vi "Generate Waveform.vi"(6 "Spl Info":cluster{"Fs":dbl, "#s":dbl}, 8 "error in":errorcluster, 9 "Wave Amp":dbl, 10 "Wave Freq":dbl, 11 "Wave Type":T1=enum."Sine" caption="Signal Type") -> (0 "error out":errorcluster, 3 "Y":waveform(dbl))   [LabVIEW 2014]
uses:
  Ctls/Wave Type.ctl
  <vilib>/measure/NI_MABase.lvlib
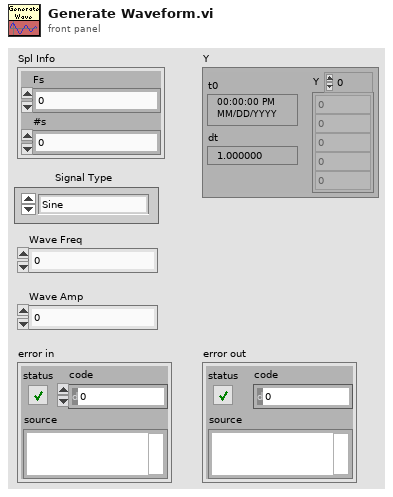
[diagram p1: front panel]
types:
  T1 = typedef "Wave Type.ctl" = enum16{"Bimodal Sine Wave", "Uniform White Noise", "Sine", "Square", "Ramp", "White Noise", "Square with Noise", "Sine with Noise"}
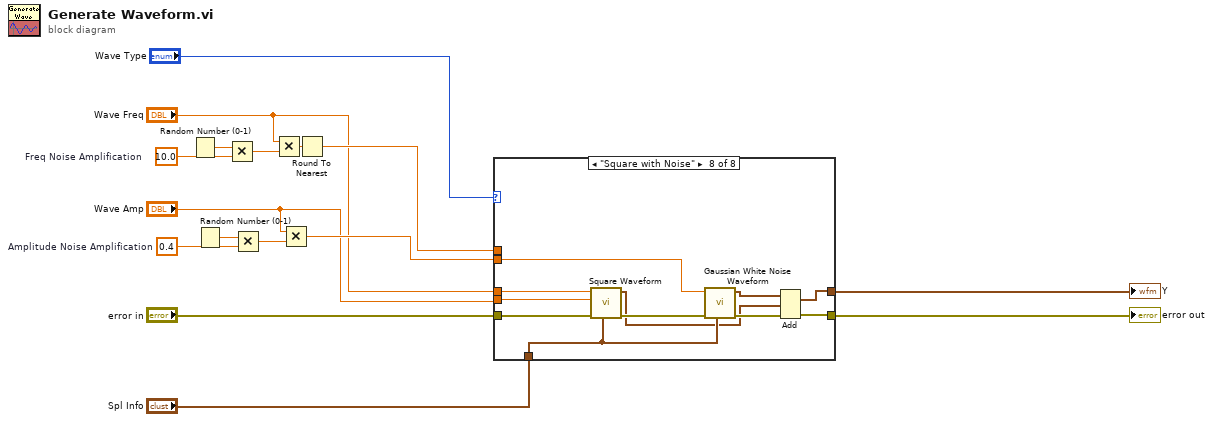
[diagram p0: block diagram]
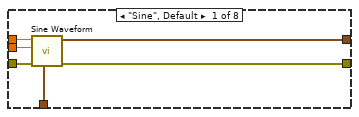
[diagram p2: hidden frame]
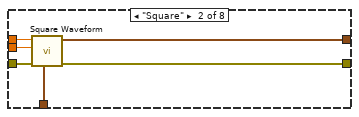
[diagram p3: hidden frame]
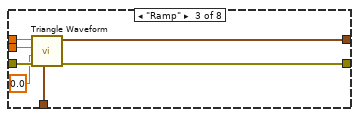
[diagram p4: hidden frame]
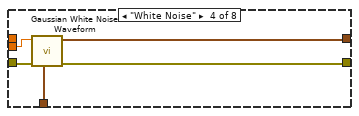
[diagram p5: hidden frame]
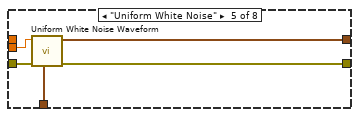
[diagram p6: hidden frame]
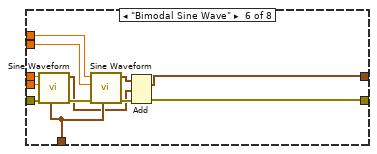
[diagram p7: hidden frame]
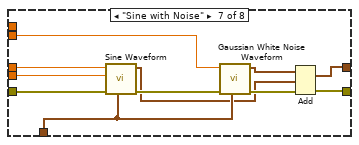
[diagram p8: hidden frame]
diagram:
  w14 = 0.4  # Amplitude Noise Amplification
  w13 = 10.0  # Freq Noise Amplification
  n1 = Random Number (0-1)() -> (number: 0 to 1=w12:dbl)
  n2 = Random Number (0-1)() -> (number: 0 to 1=w11:dbl)
  n3 = Multiply(x=w12, y=w13) -> (x*y=w15:dbl)
  n4 = Multiply(x=w11, y=w14) -> (x*y=w16:dbl)
  n5 = Multiply(x="Wave Freq", y=w15) -> (x*y=w7:dbl)
  n6 = Multiply(x="Wave Amp", y=w16) -> (x*y=w10:dbl)
  n7 = Round To Nearest(number=w7) -> (nearest integer value=w8:dbl)
  n8 = case shown="\"Square with Noise\"" "Wave Type" {
    tunnel: "Spl Info" -> [w22 w23 w30 w39 w45 w54 w65 w76]
    tunnel: "Wave Freq" -> [w21 w25 w32 _ _ w57 w68 w79]
    tunnel: "Wave Amp" -> [w20 w24 w31 w36 w41 w56 w67 w78]
    tunnel: "error in" -> [w19 w28 w35 w37 w44 w55 w66 w77]
    tunnel: [w18 w27 w34 w40 w43 w51 w62 w73] -> w4
    tunnel: [w17 w26 w33 w38 w42 w50 w61 w72] -> w5
    tunnel: w8 -> [_ _ _ _ _ w46 _ _]
    tunnel: w10 -> [_ _ _ _ _ w47 w58 w69]
    frame "Sine", Default {
      n9 = call <vilib>:"Sine Waveform.vi"("sampling info"=w22, "error in (no error)"=w19, "amplitude"=w20, "frequency"=w21) -> ("error out"=w18:errorcluster, "signal out"=w17:waveform(dbl))  [unwired: 6 in]
    }
    frame "Square" {
      n10 = call <vilib>:"Square Waveform.vi"("sampling info"=w23, "error in (no error)"=w28, "amplitude"=w24, "frequency"=w25) -> ("error out"=w27:errorcluster, "signal out"=w26:waveform(dbl))  [unwired: 6 in]
    }
    frame "Ramp" {
      n11 = call <vilib>:"Triangle Waveform.vi"("sampling info"=w30, "error in (no error)"=w35, "phase"=0.0, "amplitude"=w31, "frequency"=w32) -> ("error out"=w34:errorcluster, "signal out"=w33:waveform(dbl))  [unwired: 5 in]
    }
    frame "White Noise" {
      n12 = call <vilib>:"Gaussian White Noise Waveform.vi"("sampling info"=w39, "error in (no error)"=w37, "standard deviation"=w36) -> ("error out"=w40:errorcluster, "signal out"=w38:waveform(dbl))  [unwired: 7 in]
    }
    frame "Uniform White Noise" {
      n13 = call <vilib>:"Uniform White Noise Waveform.vi"("sampling info"=w45, "error in (no error)"=w44, "amplitude"=w41) -> ("error out"=w43:errorcluster, "signal out"=w42:waveform(dbl))  [unwired: 7 in]
    }
    frame "Bimodal Sine Wave" {
      n14 = call <vilib>:"Sine Waveform.vi"("sampling info"=w54, "error in (no error)"=w55, "amplitude"=w56, "frequency"=w57) -> ("error out"=w53:errorcluster, "signal out"=w48:waveform(dbl))  [unwired: 6 in]
      n15 = call <vilib>:"Sine Waveform.vi"("sampling info"=w54, "error in (no error)"=w53, "amplitude"=w47, "frequency"=w46) -> ("error out"=w52:errorcluster, "signal out"=w49:waveform(dbl))  [unwired: 6 in]
      n16 = Add(1:w48, 2:w49, 4:w52) -> (0:w50:waveform(dbl), 3:w51:errorcluster)
    }
    frame "Sine with Noise" {
      n17 = call <vilib>:"Sine Waveform.vi"("sampling info"=w65, "error in (no error)"=w66, "amplitude"=w67, "frequency"=w68) -> ("error out"=w64:errorcluster, "signal out"=w59:waveform(dbl))  [unwired: 6 in]
      n18 = call <vilib>:"Gaussian White Noise Waveform.vi"("sampling info"=w65, "error in (no error)"=w64, "standard deviation"=w58) -> ("error out"=w63:errorcluster, "signal out"=w60:waveform(dbl))  [unwired: 7 in]
      n19 = Add(1:w59, 2:w60, 4:w63) -> (0:w61:waveform(dbl), 3:w62:errorcluster)
    }
    frame "Square with Noise" {
      n20 = call <vilib>:"Square Waveform.vi"("sampling info"=w76, "error in (no error)"=w77, "amplitude"=w78, "frequency"=w79) -> ("error out"=w75:errorcluster, "signal out"=w70:waveform(dbl))  [unwired: 6 in]
      n21 = call <vilib>:"Gaussian White Noise Waveform.vi"("sampling info"=w76, "error in (no error)"=w75, "standard deviation"=w69) -> ("error out"=w74:errorcluster, "signal out"=w71:waveform(dbl))  [unwired: 7 in]
      n22 = Add(1:w70, 2:w71, 4:w74) -> (0:w72:waveform(dbl), 3:w73:errorcluster)
    }
  }
  "Y" <- w5
  "error out" <- w4
